vi "StopAndAcquire.vi"() -> ()   [LabVIEW 2016]
uses:
  <vilib>/Utility/file.llb/Write Delimited Spreadsheet (DBL).vi
panel:
  out "error in (no error)":errorcluster
  in  "Run":bool=TRUE
  in  "即将记录":i32
  in  "osc":refnum<visa-resource-name>
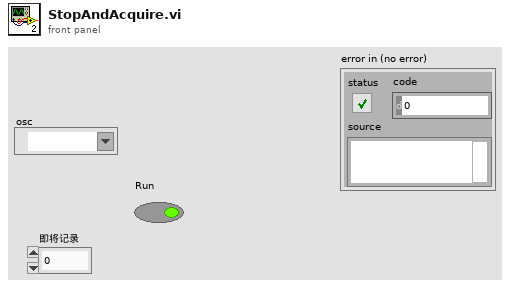
[diagram p1: front panel]
types:
  T1 = typedef "NI_Matrix.lvlib/RealMatrix.ctl" = dbl[][]
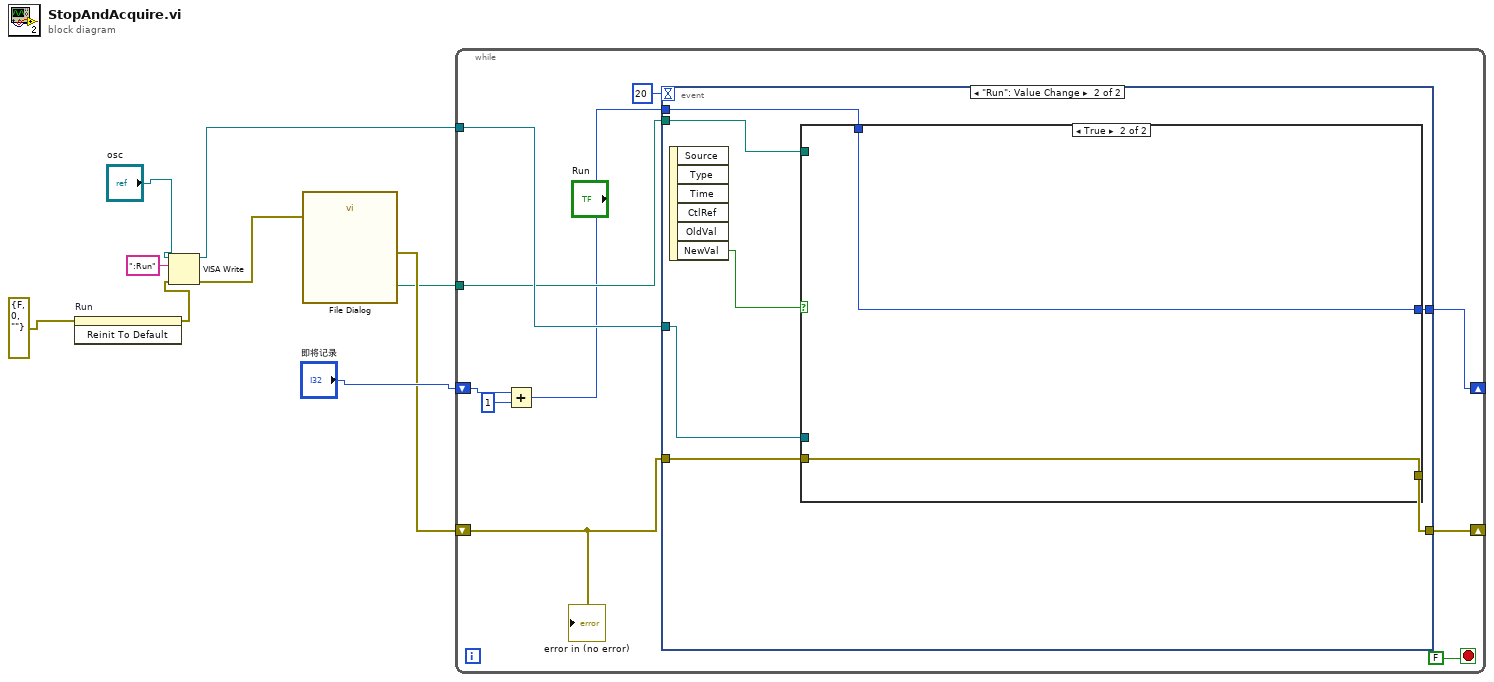
[diagram p0: block diagram]
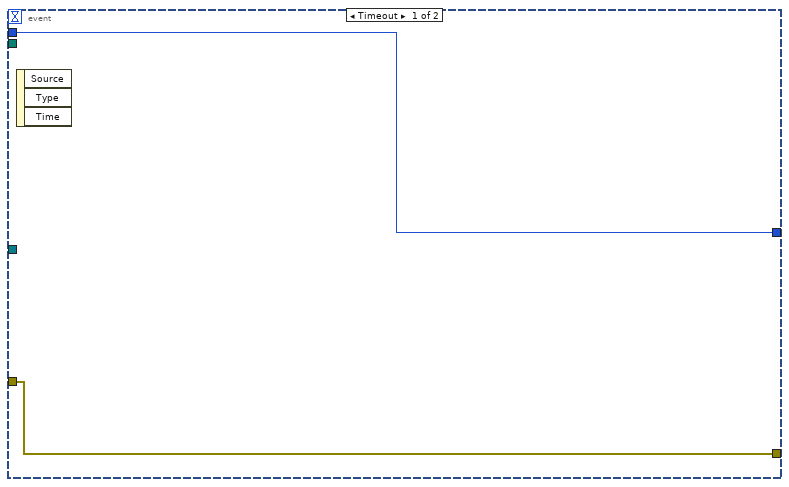
[diagram p2: hidden frame]
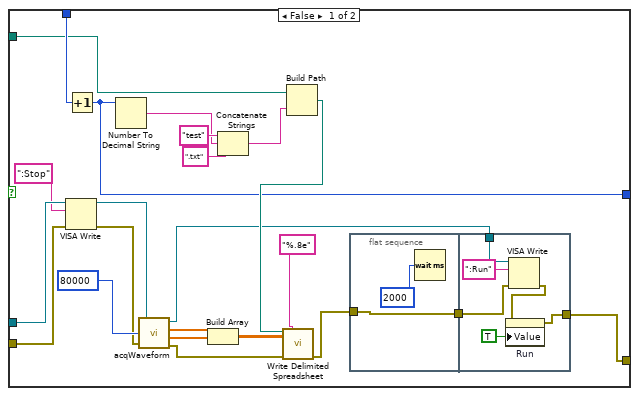
[diagram p3: hidden frame]
diagram:
  n1 = invoke on="Run" class="Bool (strict)" method="Reinit To Default"(error in=errorcluster {"status"=FALSE, "code"=0, "source"=""} ("error in (no error)")) -> (error out=w5:errorcluster)  [unwired: 2 in, 2 out]
  n2 = VISA Write(VISA resource name="osc", write buffer=":Run", error in (no error)=w5) -> (VISA resource name out=w4:refnum<visa-resource-name>, error out=w3:errorcluster)  [unwired: 1 out]
  n3 = call "File Dialog"("error in"=w3) -> ("selected path"=w1:path, "error out"=w2:errorcluster)  [unwired: 11 in, 2 out]
  n4 = while {
    shift-right: [w17] -> _
    shift-left: w2 -> [w18]
    tunnel: w4 -> [w16]
    tunnel: w1 -> [w15]
    shift-right: [w11] -> _
    shift-left: "即将记录" -> [w14]
    stop <- FALSE stop-if-true
    n5 = Add(x=w14, y=1) -> (x+y=w12:i32)
    n6 = event shown="[1] \"Run\": Value Change" {
      selector: _ -> [_ _]
      dyn-events: _ -> [_ _]
      timeout: 20 -> [_ _]
      tunnel: w16 -> [_ w26]
      tunnel: w18 -> [w21 w27]
      tunnel: [w21 w25] -> w17
      tunnel: w15 -> [_ w23]
      tunnel: w12 -> [w20 w24]
      tunnel: [w20 w22] -> w11
      event Timeout {
        n7 = event-data() -> ()  [unwired: 1 in, 3 out]
      }
      event "Run": Value Change {
        n8 = event-data() -> ("NewVal"=w28:bool)  [unwired: 1 in, 5 out]
        n9 = case shown="True" w28 {
          tunnel: w27 -> [w35 w61]
          tunnel: w26 -> [w37 _]
          tunnel: [w30 w61] -> w25
          tunnel: w24 -> [w45 w60]
          tunnel: w23 -> [w41 _]
          tunnel: [w29 w60] -> w22
          frame False {
            n10 = VISA Write(VISA resource name=w37, write buffer=":Stop", error in (no error)=w35) -> (VISA resource name out=w33:refnum<visa-resource-name>, error out=w34:errorcluster)  [unwired: 1 out]
            n11 = Increment(x=w45) -> (x+1=w29:i32)
            n12 = Number To Decimal String(number=w29) -> (decimal integer string=w43:string)  [unwired: 1 in]
            n13 = call "acqWaveform.vi"("OSC in"=w33, "Points"=u32 80000, "error in (no error)"=w34) -> ("OSC out"=w32:refnum<visa-resource-name>, "time sequence"=w50:dbl[], "Voltage sequence"=w49:dbl[], "error out"=w46:errorcluster)
            n14 = Build Array(w50, w49) -> (w48:T1)
            n15 = Concatenate Strings("test" ("string"), w43, ".txt" ("string")) -> (w40:string)
            n16 = Build Path(base path=w41, name or relative path=w40) -> (appended path=w39:path)
            n17 = call-poly <vilib>:"Write Delimited Spreadsheet.vi"("file path (dialog if empty)"=w39, "format (%.3f)"="%.8e", "2D data"=w48, "error in (no error)"=w46) -> ("error out"=w38:errorcluster)  [unwired: 10 in, 1 out]
            n18 = flat-sequence {
              tunnel: w38 -> [w52]
              tunnel: [w52] -> w31
              tunnel: w32 -> [w59]
              tunnel: w31 -> [w57]
              tunnel: [w54] -> w30
              frame #0 {
                n19 = Wait (ms)(milliseconds to wait=u32 2000) -> ()  [unwired: 1 out]
              }
              frame #1 {
                n20 = VISA Write(VISA resource name=w59, write buffer=":Run", error in (no error)=w57) -> (error out=w55:errorcluster)  [unwired: 2 out]
                n21 = property on="Run" class="Bool (strict)"(error in=w55, "Value"=TRUE ("Run")) -> (error out=w54:errorcluster)  [unwired: 1 in, 1 out]
              }
            }
          }
          frame True {
          }
        }
      }
    }
    "error in (no error)" <- w18
  }
